vi "SQL Server Execute (test).vi"() -> ()   [LabVIEW 2010]
doc: "The BIMS_Collector.UDL universal data link file for connecting to the AFS_Ballistics SQL Server DB is located in the BIMS Collector project folder. It is configured to attach to the ICELA_DV instance of SQL Server 2005 on the ESTS03 file server in E320."
uses:
  <vilib>/addons/database/Connection.llb/DB Tools Open Connec (Path).vi
  <vilib>/addons/database/Connection.llb/Conn Execute.vi
  <vilib>/addons/database/Recordset.llb/Rec Fetch Recordset Data (R).vi
  <vilib>/addons/database/Recordset.llb/Rec Destroy - Connection.vi
  <vilib>/addons/database/NI_Database_API.lvlib
panel:
  in  "SQL Statement":string
  out "recordset data":variant[][](array[variant])
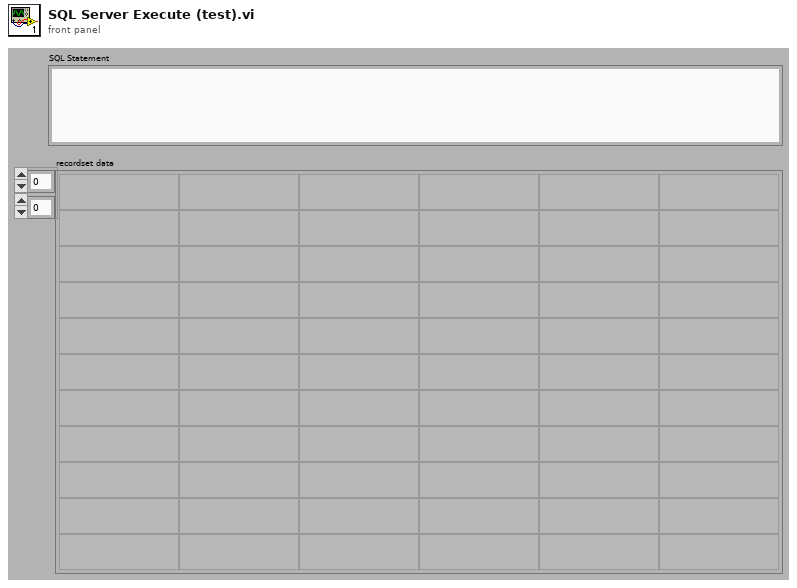
[diagram p1: front panel]
types:
  T1 = typedef "NI_Database_API.lvlib/Conn ObjectReference.ctl" = refnum<k1>
  T2 = typedef "NI_Database_API.lvlib/Rec ObjectReference.ctl" = refnum<k1>
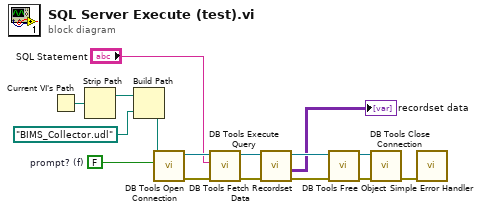
[diagram p0: block diagram]
diagram:
  w16 = FALSE  # prompt? (f)
  n1 = Current VI's Path() -> (path=w4:path)
  n2 = Strip Path(path=w4) -> (stripped path=w3:path)  [unwired: 1 out]
  n3 = Build Path(base path=w3, name or relative path=path "BIMS_Collector.udl" ("connectString")) -> (appended path=w1:path)
  n4 = call-poly <vilib>:"DB Tools Open Connection.vi"("prompt? (F)"=w16, "connection information"=w1) -> ("error out"=w8:errorcluster, "connection reference"=w15:T1)  [unwired: 6 in]
  n5 = call-poly <vilib>:"DB Tools Execute Query.vi"("error in (no error)"=w8, "SQL query"="SQL Statement", "connection reference"=w15) -> ("error out"=w9:errorcluster, "recordset reference"=w14:T2)  [unwired: 5 in]
  n6 = call-poly <vilib>:"DB Tools Fetch Recordset Data.vi"("error in (no error)"=w9, "recordset reference"=w14) -> ("error out"=w10:errorcluster, "recordset data"=→"recordset data":variant[][], "recordset reference out"=w13:T2)  [unwired: 3 in]
  n7 = call-poly <vilib>:"DB Tools Free Object.vi"("error in (no error)"=w10, "recordset reference"=w13) -> ("error out"=w11:errorcluster, "connection reference"=w12:T1)  [unwired: 8 in]
  n8 = call <vilib>:"DB Tools Close Connection.vi"("error in (no error)"=w11, "connection reference"=w12) -> ("error out"=w7:errorcluster)  [unwired: 5 in]
  n9 = call <vilib>:"Simple Error Handler.vi"("error in (no error)"=w7) -> ()  [unwired: 4 in, 5 out]
